vi "Set Routing Channel State-Value Table.vi"(8 "error in":errorcluster, 9 "state values":i32[](array[numeric]), 10 "state names":string[](array[string]), 11 "routing channel in":T1 format="%.0x") -> (0 "error out":errorcluster, 3 "routing channel out":T1=18446744073709551615 format="%.0x")   [LabVIEW 2017, in "Routing and Faulting Scripting.lvlib"]
uses:
  Routing and Faulting Scripting.lvlib
  <vilib>/NI Veristand/Custom Device API/Custom Device Item Ref.ctl
  NationalInstruments.VeriStand.SystemDefinitionAPI
  NationalInstruments.VeriStand.SystemStorage
  <vilib>/NI Veristand/Custom Device API/Custom Device API.lvlib
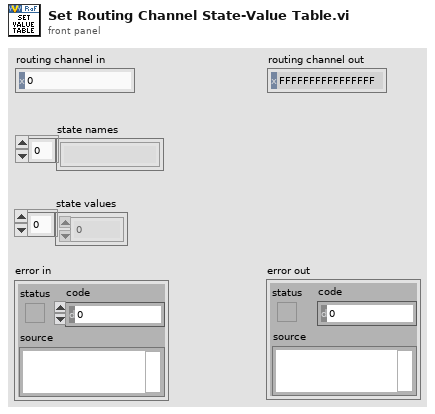
[diagram p1: front panel]
types:
  T1 = typedef "Custom Device API.lvlib/Custom Device Item Ref.ctl" = u64
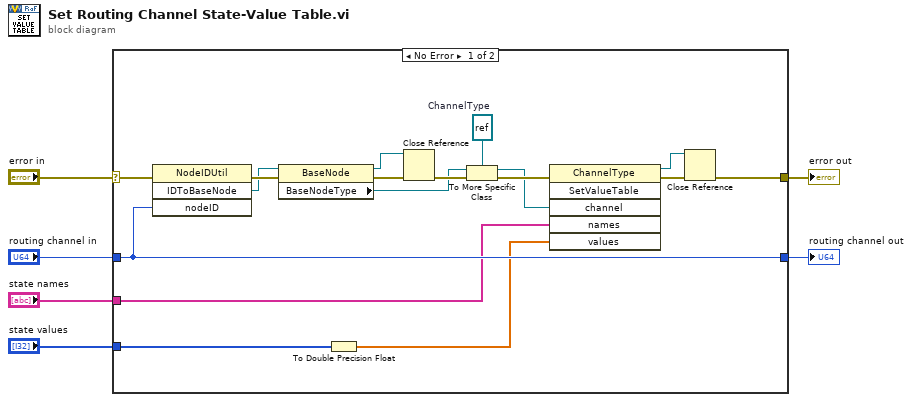
[diagram p0: block diagram]
diagram:
  n1 = case shown="No Error" "error in" {
    selector: "error in" -> [w20 w25]
    tunnel: [w19 w25] -> w5
    tunnel: "routing channel in" -> [w18 w24]
    tunnel: [w18 w24] -> w3
    tunnel: "state names" -> [w10 _]
    tunnel: "state values" -> [w9 _]
    frame No Error {
      w16 = refnum<k24> refnum  # ChannelType
      n2 = invoke class="NodeIDUtil" method="IDToBaseNode"(error in=w20, "nodeID"=w18) -> (error out=w23:errorcluster, "IDToBaseNode"=w21:refnum<k24>)  [unwired: 2 in, 2 out]
      n3 = property class="BaseNode"(reference=w21, error in=w23) -> (reference out=w8:refnum<k24>, error out=w22:errorcluster, "BaseNodeType"=w13:refnum<k24>)
      n4 = To Double Precision Float(number=w9) -> (double precision float=w7:dbl[])
      n5 = Close Reference(reference=w8, error in (no error)=w22) -> (error out=w14:errorcluster)
      n6 = To More Specific Class(target class=w16, reference=w13, error in=w14) -> (specific class reference=w15:refnum<k24>, error out=w17:errorcluster)
      n7 = invoke class="ChannelType" method="SetValueTable"(error in=w17, "channel"=w15, "names"=w10, "values"=w7) -> (reference out=w11:refnum<k24>, error out=w12:errorcluster)  [unwired: 2 in, 4 out]
      n8 = Close Reference(reference=w11, error in (no error)=w12) -> (error out=w19:errorcluster)
    }
    frame Error {
    }
  }
  "routing channel out" <- w3
  "error out" <- w5
